vi "messages.vi"() -> ()   [LabVIEW 2014]
uses:
  Controls/TCP State Machine States.ctl
panel:
  in  "Devices":i32
  in  "New Command":string
  in  "New Message":string
  in  "TCP State Machine States":T1
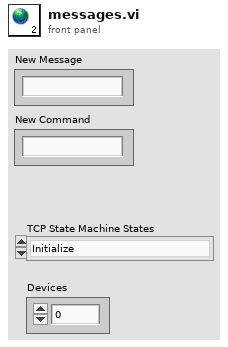
[diagram p1: front panel]
types:
  T1 = typedef "TCP State Machine States.ctl" = enum16{"Initialize", "Status Check", "Read Data", "Stop"}
diagram:
